vi "GetMicronArgs.vi"(8 "error in (no error)":errorcluster, 10 "Args":string[](array[string]), 11 "Default Connection String":string="localhost:50051") -> (0 "error out":errorcluster, 3 "Micron Args":T1)   [LabVIEW 2019, in "MicronServer.lvlib" / "ServiceBase.lvclass"]
uses:
  ServiceBase.lvclass
  Typedefs/Micron Args.ctl
  <vilib>/Wiresmith Technology/G CLI/Argument Parser/Option Class/Option Configuration.ctl
  <vilib>/Wiresmith Technology/G CLI/Argument Parser/Option Class/Argument Type.ctl
  <vilib>/SLL Toolkit/SLL String/_SubVIs/String to 1D String Array.vi
  <vilib>/SLL Toolkit/SLL String/_SubVIs/String to I32.vi
  <vilib>/Wiresmith Technology/G CLI/Argument Parser/Option Set Class/Option Set.lvclass
  <vilib>/Wiresmith Technology/G CLI/Argument Parser/Option Class/Option.lvclass
  <vilib>/SLL Toolkit/SLL String/SLL String.lvlib
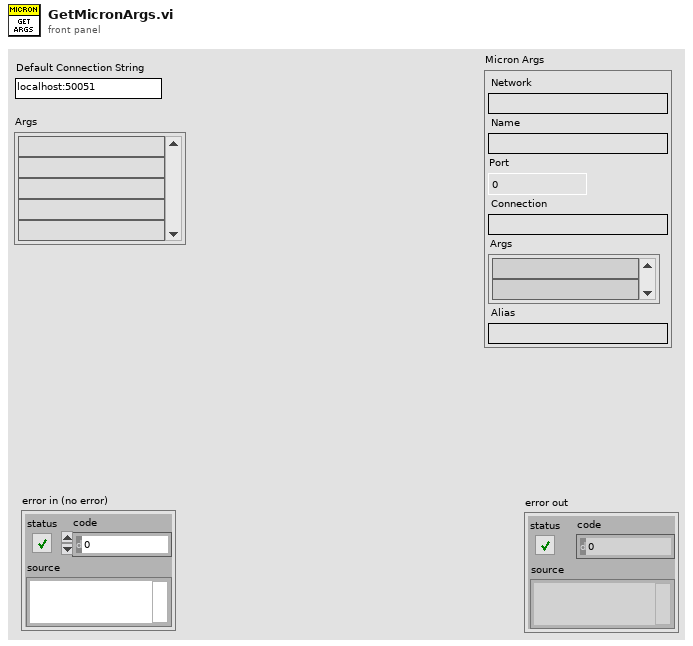
[diagram p1: front panel]
types:
  T1 = typedef "MicronServer.lvlib/ServiceBase.lvclass/Micron Args.ctl" = cluster{"Network":string, "Name":string, "Port":i32, "Connection":string, "Args":string[], "Alias":string}
  T2 = typedef "Option Parser.lvlib/Option.lvclass/Argument Type.ctl" = enum16{"flag", "value"}
  T3 = typedef "Option Parser.lvlib/Option.lvclass/Option Configuration.ctl" = cluster{"Option Type":T2, "Option Labels":string[], "Key":string, "Description":string, "Required":bool, "Default Value":string}
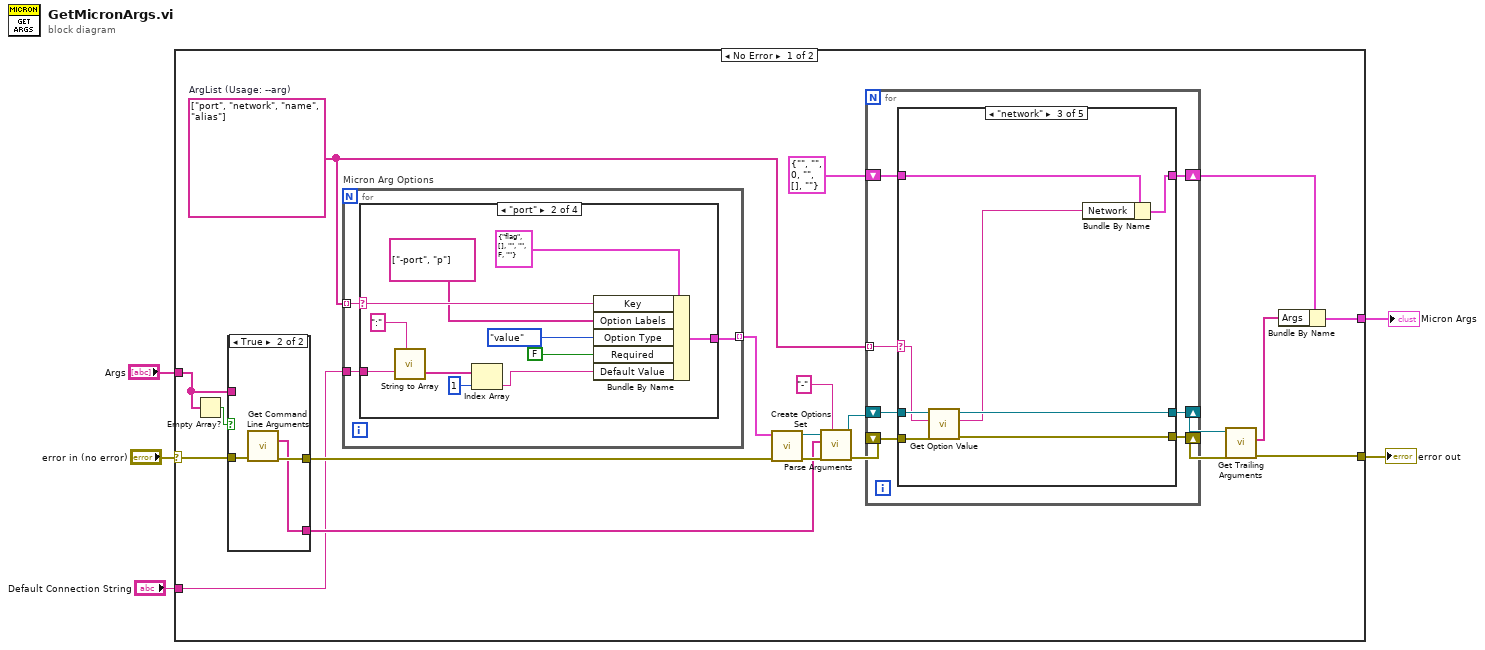
[diagram p0: block diagram]
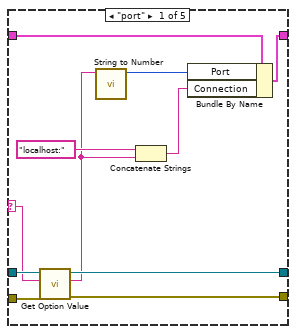
[diagram p3: hidden frame]
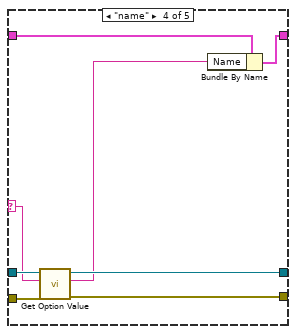
[diagram p5: hidden frame]
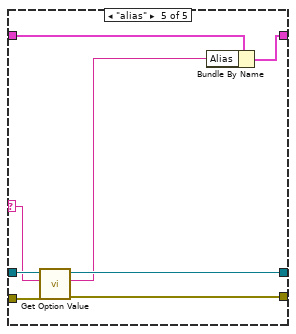
[diagram p6: hidden frame]
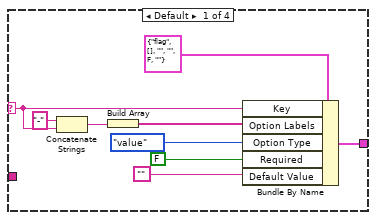
[diagram p7: hidden frame]
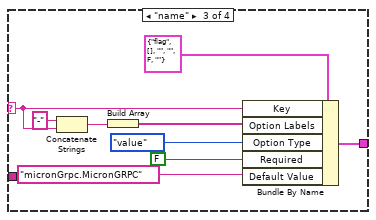
[diagram p8: hidden frame]
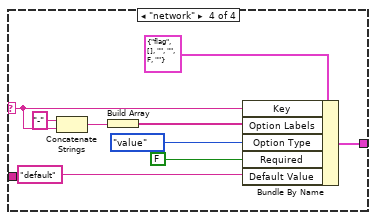
[diagram p9: hidden frame]
diagram:
  n1 = case shown="No Error" "error in (no error)" {
    selector: "error in (no error)" -> [w25 w117]
    tunnel: [w11 w117] -> w4
    tunnel: [w13 _] -> w3
    tunnel: "Args" -> [w7 _]
    tunnel: "Default Connection String" -> [w6 _]
    frame No Error {
      w18 = string[] ["port", "network", "name", "alias"]  # ArgList (Usage: --arg)
      n2 = Empty Array?(array=w7) -> (empty?=w8:bool)
      n3 = case shown="True" w8 {
        tunnel: w25 -> [w26 w30]
        tunnel: [w26 w29] -> w20
        tunnel: [w27 w28] -> w9
        tunnel: w7 -> [w27 _]
        frame False {
        }
        frame True {
          n4 = call <vilib>:"Get Command Line Arguments.vi"("error in (no error)"=w30) -> ("error out"=w29:errorcluster, "arguments"=w28:string[])  [unwired: 8 in, 1 out]
        }
      }
      n5 = for "Micron Arg Options" {
        tunnel: w18 -> [w78] mode=indexing
        tunnel: [w77] -> w19 mode=indexing
        tunnel: w6 -> [w76]
        n6 = case shown="\"port\"" w78 {
          selector: w78 -> [w80 w94 w101 w110]
          tunnel: [w86 w97 w106 w115] -> w77
          tunnel: w76 -> [_ w92 _ _]
          frame Default {
            n7 = Concatenate Strings("-" ("string"), w80) -> (w81:string)
            n8 = Build Array(w81) -> (w85:string[])
            n9 = Bundle By Name(cluster=T3 {"Option Type"=enum."flag", "Option Labels"=[], "Key"="", "Description"="", "Required"=FALSE, "Default Value"=""} ("Option Config"), "Key"=w80, "Option Labels"=w85, "Option Type"=Argument_Type."value", "Required"=FALSE, "Default Value"="") -> (w86:T3)
          }
          frame "port" {
            n10 = call-poly <vilib>:"String to Array.vi"("Delimiter (,)"=":", "String"=w92) -> ("Array[]"=w90:string[])  [unwired: 6 in]
            n11 = Index Array(array=w90, index=1) -> (element=w88:string)
            n12 = Bundle By Name(cluster=T3 {"Option Type"=enum."flag", "Option Labels"=[], "Key"="", "Description"="", "Required"=FALSE, "Default Value"=""} ("Option Config"), "Key"=w94, "Option Labels"=string[] ["-port", "p"], "Option Type"=Argument_Type."value", "Required"=FALSE, "Default Value"=w88) -> (w97:T3)
          }
          frame "name" {
            n13 = Concatenate Strings("-" ("string"), w101) -> (w102:string)
            n14 = Build Array(w102) -> (w105:string[])
            n15 = Bundle By Name(cluster=T3 {"Option Type"=enum."flag", "Option Labels"=[], "Key"="", "Description"="", "Required"=FALSE, "Default Value"=""} ("Option Config"), "Key"=w101, "Option Labels"=w105, "Option Type"=Argument_Type."value", "Required"=FALSE, "Default Value"="micronGrpc.MicronGRPC") -> (w106:T3)
          }
          frame "network" {
            n16 = Concatenate Strings("-" ("string"), w110) -> (w111:string)
            n17 = Build Array(w111) -> (w114:string[])
            n18 = Bundle By Name(cluster=T3 {"Option Type"=enum."flag", "Option Labels"=[], "Key"="", "Description"="", "Required"=FALSE, "Default Value"=""} ("Option Config"), "Key"=w110, "Option Labels"=w114, "Option Type"=Argument_Type."value", "Required"=FALSE, "Default Value"="default") -> (w115:T3)
          }
        }
      }
      n19 = call <vilib>:"Create Options Set.vi"("error in (no error)"=w20, "Options"=w19) -> ("error out"=w24:errorcluster, "Option Set out"=w23:refnum<class "Option Set.lvclass">)  [unwired: 8 in]
      n20 = call <vilib>:"Parse Arguments.vi"("Label Marker (-)"="-", "error in (no error)"=w24, "Arguments"=w9, "Option Set in"=w23) -> ("error out"=w21:errorcluster, "Option Set out"=w22:refnum<class "Option Set.lvclass">)  [unwired: 4 in, 2 out]
      n21 = for {
        shift-right: [w35] -> w15
        shift-left: w22 -> [w37]
        shift-right: [w34] -> w16
        shift-left: w21 -> [w36]
        tunnel: w18 -> [w33] mode=indexing
        shift-right: [w31] -> w14
        shift-left: T1 {"Network"="", "Name"="", "Port"=0, "Connection"="", "Args"=[], "Alias"=""} ("Micron Args") -> [w32]
        n22 = case shown="\"network\"" w33 {
          selector: w33 -> [w44 _ w55 w63 w71]
          tunnel: w37 -> [w48 w50 w59 w67 w75]
          tunnel: w36 -> [w47 w49 w58 w66 w74]
          tunnel: [w46 w50 w57 w65 w73] -> w35
          tunnel: [w45 w49 w56 w64 w72] -> w34
          tunnel: w32 -> [w43 w51 w54 w62 w70]
          tunnel: [w42 w51 w53 w61 w69] -> w31
          frame "port" {
            n23 = call <vilib>:"Get Option Value.vi"("error in (no error)"=w47, "Option Key"=w44, "Option Set in"=w48) -> ("error out"=w45:errorcluster, "Value"=w39:string, "Option Set out"=w46:refnum<class "Option Set.lvclass">)  [unwired: 5 in, 1 out]
            n24 = call-poly <vilib>:"String to Number.vi"("String"=w39) -> ("Numeric"=w41:i32)  [unwired: 10 in]
            n25 = Concatenate Strings("localhost:" ("string"), w39) -> (w38:string)
            n26 = Bundle By Name(cluster=w43, "Port"=w41, "Connection"=w38) -> (w42:T1)
          }
          frame Default {
          }
          frame "network" {
            n27 = call <vilib>:"Get Option Value.vi"("error in (no error)"=w58, "Option Key"=w55, "Option Set in"=w59) -> ("error out"=w56:errorcluster, "Value"=w52:string, "Option Set out"=w57:refnum<class "Option Set.lvclass">)  [unwired: 5 in, 1 out]
            n28 = Bundle By Name(cluster=w54, "Network"=w52) -> (w53:T1)
          }
          frame "name" {
            n29 = call <vilib>:"Get Option Value.vi"("error in (no error)"=w66, "Option Key"=w63, "Option Set in"=w67) -> ("error out"=w64:errorcluster, "Value"=w60:string, "Option Set out"=w65:refnum<class "Option Set.lvclass">)  [unwired: 5 in, 1 out]
            n30 = Bundle By Name(cluster=w62, "Name"=w60) -> (w61:T1)
          }
          frame "alias" {
            n31 = call <vilib>:"Get Option Value.vi"("error in (no error)"=w74, "Option Key"=w71, "Option Set in"=w75) -> ("error out"=w72:errorcluster, "Value"=w68:string, "Option Set out"=w73:refnum<class "Option Set.lvclass">)  [unwired: 5 in, 1 out]
            n32 = Bundle By Name(cluster=w70, "Alias"=w68) -> (w69:T1)
          }
        }
      }
      n33 = call <vilib>:"Get Trailing Arguments.vi"("error in (no error)"=w16, "Option Set in"=w15) -> ("error out"=w11:errorcluster, "Arguments"=w12:string[])  [unwired: 7 in, 1 out]
      n34 = Bundle By Name(cluster=w14, "Args"=w12) -> (w13:T1)
    }
    frame Error {
    }
  }
  "error out" <- w4
  "Micron Args" <- w3
